vi "Beam_and_Cathode.vi"() -> ()   [LabVIEW 2018]
panel:
  out "?":string
  out "?":string
  out "?":string
  out "?":string
  out "?":string
  out "?":string
  in  "Set Operate Temp C":bool
  out "?":string
  out "?":bool
  out "?":bool
  in  "Set Warm Temp C":bool
  out "?":string
  out "?":string
  out "?":bool
  out "?":bool
  in  "Set Operate Temp B":bool
  out "?":string
  out "?":bool
  out "?":bool
  in  "Set Warm Temp B":bool
  out "?":string
  out "?":string
  out "?":bool
  out "?":bool
  in  "Set Operate Temp A":bool
  out "?":string
  out "?":bool
  out "?":bool
  in  "Set Warm Temp A":bool
  out "?":string
  out "?":string
  out "?":bool
  out "?":bool
  out "Cathode C":string
  out "Cathode B":string
  out "?":string
  out "?":bool
  out "?":bool
  out "?":string
  out "?":bool
  out "?":bool
  out "Cathode A":string
  out "?":string
  out "?":bool
  out "?":bool
  out "?":string
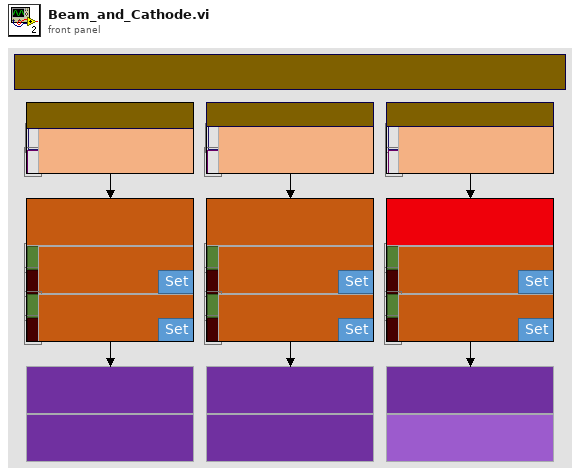
[diagram p1: front panel]
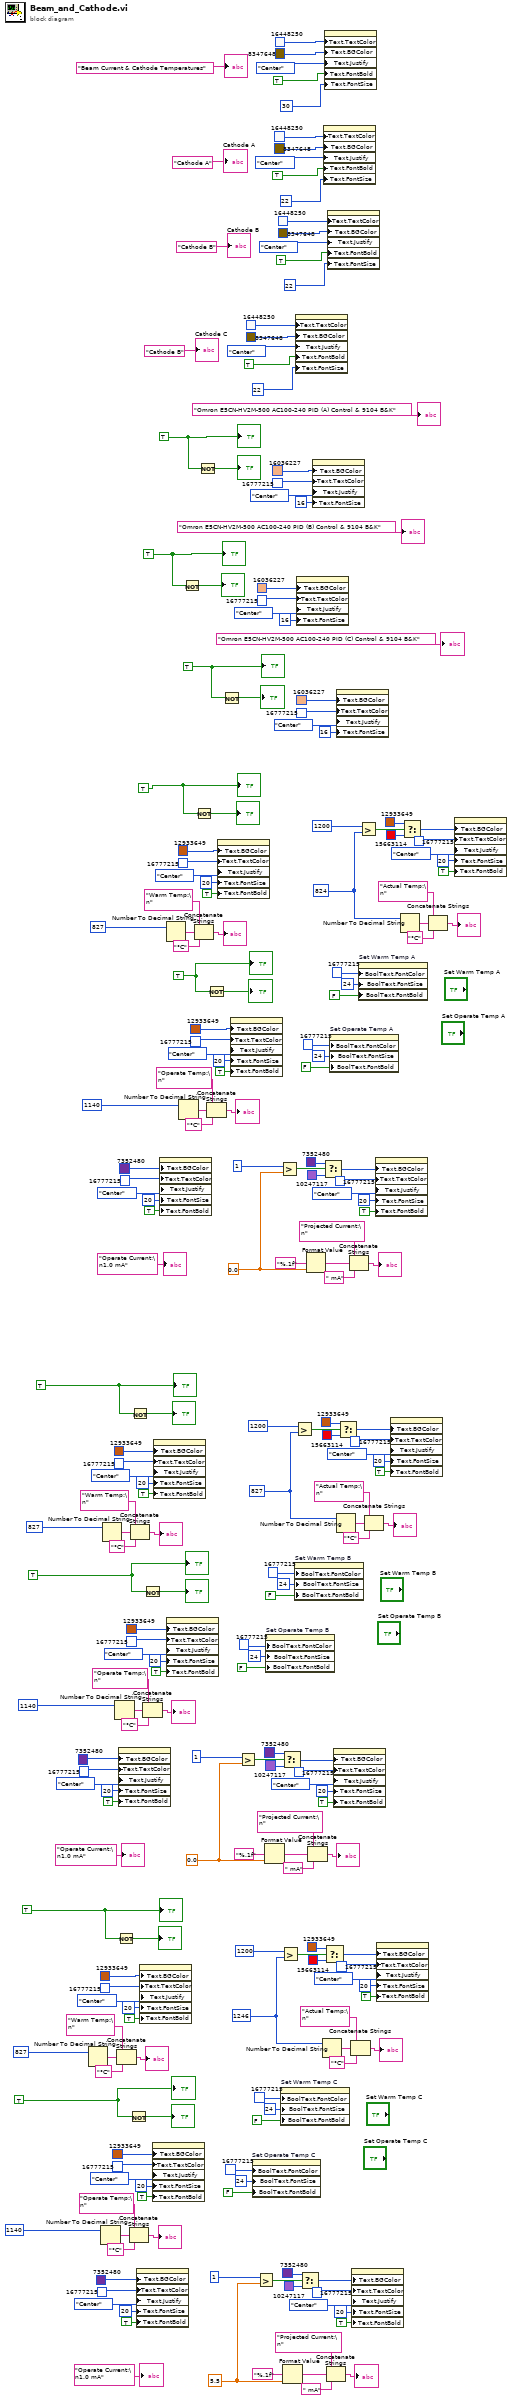
[diagram p0: block diagram]
diagram:
  w1 = 5.5
  w22 = 0.0
  w43 = 0.0
  w64 = TRUE
  w66 = TRUE
  w67 = 1246 ("number")
  w108 = TRUE
  w110 = TRUE
  w111 = 827 ("number")
  w152 = TRUE
  w154 = TRUE
  w155 = 824 ("number")
  w198 = TRUE
  w204 = TRUE
  w211 = TRUE
  n1 = Number To Decimal String(number=827) -> (decimal integer string=w92:string)  [unwired: 1 in]
  n2 = Number To Decimal String(number=1140) -> (decimal integer string=w79:string)  [unwired: 1 in]
  n3 = Number To Decimal String(number=827) -> (decimal integer string=w136:string)  [unwired: 1 in]
  n4 = Number To Decimal String(number=1140) -> (decimal integer string=w123:string)  [unwired: 1 in]
  n5 = Not(x=w64) -> (.not. x?=→"?":bool)
  n6 = Concatenate Strings("Warm Temp:\n", w92, "°C" ("string")) -> (→"?":string)
  n7 = property class="Str"("Text.BGColor"=u32 7352480, "Text.TextColor"=u32 16777215, "Text.Justify"=enum16{"Left", "Center", "Right"}."Center" ("Text.Justification"), "Text.FontSize"=u32 20 ("Text.Font:Size"), "Text.FontBold"=TRUE ("Text.Font:Bold")) -> ()  [unwired: 2 in, 2 out]
  n8 = Not(x=w66) -> (.not. x?=→"?":bool)
  n9 = Concatenate Strings("Operate Temp:\n", w79, "°C" ("string")) -> (→"?":string)
  n10 = Not(x=w108) -> (.not. x?=→"?":bool)
  n11 = Concatenate Strings("Warm Temp:\n", w136, "°C" ("string")) -> (→"?":string)
  n12 = property class="Str"("Text.BGColor"=u32 7352480, "Text.TextColor"=u32 16777215, "Text.Justify"=enum16{"Left", "Center", "Right"}."Center" ("Text.Justification"), "Text.FontSize"=u32 20 ("Text.Font:Size"), "Text.FontBold"=TRUE ("Text.Font:Bold")) -> ()  [unwired: 2 in, 2 out]
  n13 = property class="Str"("Text.BGColor"=u32 12933649, "Text.TextColor"=u32 16777215, "Text.Justify"=enum16{"Left", "Center", "Right"}."Center" ("Text.Justification"), "Text.FontSize"=u32 20 ("Text.Font:Size"), "Text.FontBold"=TRUE ("Text.Font:Bold")) -> ()  [unwired: 2 in, 2 out]
  n14 = Not(x=w110) -> (.not. x?=→"?":bool)
  n15 = Concatenate Strings("Operate Temp:\n", w123, "°C" ("string")) -> (→"?":string)
  n16 = property class="Str"("Text.BGColor"=u32 12933649, "Text.TextColor"=u32 16777215, "Text.Justify"=enum16{"Left", "Center", "Right"}."Center" ("Text.Justification"), "Text.FontSize"=u32 20 ("Text.Font:Size"), "Text.FontBold"=TRUE ("Text.Font:Bold")) -> ()  [unwired: 2 in, 2 out]
  n17 = property class="Str"("Text.BGColor"=u32 12933649, "Text.TextColor"=u32 16777215, "Text.Justify"=enum16{"Left", "Center", "Right"}."Center" ("Text.Justification"), "Text.FontSize"=u32 20 ("Text.Font:Size"), "Text.FontBold"=TRUE ("Text.Font:Bold")) -> ()  [unwired: 2 in, 2 out]
  n18 = property class="Str"("Text.BGColor"=u32 7352480, "Text.TextColor"=u32 16777215, "Text.Justify"=enum16{"Left", "Center", "Right"}."Center" ("Text.Justification"), "Text.FontSize"=u32 20 ("Text.Font:Size"), "Text.FontBold"=TRUE ("Text.Font:Bold")) -> ()  [unwired: 2 in, 2 out]
  n19 = Number To Decimal String(number=827) -> (decimal integer string=w181:string)  [unwired: 1 in]
  n20 = property class="Str"("Text.BGColor"=u32 12933649, "Text.TextColor"=u32 16777215, "Text.Justify"=enum16{"Left", "Center", "Right"}."Center" ("Text.Justification"), "Text.FontSize"=u32 20 ("Text.Font:Size"), "Text.FontBold"=TRUE ("Text.Font:Bold")) -> ()  [unwired: 2 in, 2 out]
  n21 = Number To Decimal String(number=1140) -> (decimal integer string=w168:string)  [unwired: 1 in]
  n22 = Not(x=w204) -> (.not. x?=→"?":bool)
  n23 = Not(x=w152) -> (.not. x?=→"?":bool)
  n24 = Concatenate Strings("Warm Temp:\n", w181, "°C" ("string")) -> (→"?":string)
  n25 = Not(x=w211) -> (.not. x?=→"?":bool)
  n26 = Not(x=w154) -> (.not. x?=→"?":bool)
  n27 = Concatenate Strings("Operate Temp:\n", w168, "°C" ("string")) -> (→"?":string)
  n28 = property class="Str"("Text.BGColor"=u32 12933649, "Text.TextColor"=u32 16777215, "Text.Justify"=enum16{"Left", "Center", "Right"}."Center" ("Text.Justification"), "Text.FontSize"=u32 20 ("Text.Font:Size"), "Text.FontBold"=TRUE ("Text.Font:Bold")) -> ()  [unwired: 2 in, 2 out]
  n29 = Not(x=w198) -> (.not. x?=→"?":bool)
  n30 = property class="Str"("Text.BGColor"=u32 12933649, "Text.TextColor"=u32 16777215, "Text.Justify"=enum16{"Left", "Center", "Right"}."Center" ("Text.Justification"), "Text.FontSize"=u32 20 ("Text.Font:Size"), "Text.FontBold"=TRUE ("Text.Font:Bold")) -> ()  [unwired: 2 in, 2 out]
  n31 = Greater?(x=1, y=w22) -> (0:w27:bool)
  n32 = property on="Set Operate Temp C" class="Bool (strict)"("BoolText.FontColor"=u32 16777215, "BoolText.FontSize"=u32 24 ("Boolean Text.Font:Size"), "BoolText.FontBold"=FALSE ("Boolean Text.Font:Bold")) -> ()  [unwired: 2 in, 2 out]
  n33 = Greater?(x=1, y=w1) -> (0:w6:bool)
  n34 = Format Value(format string="%.1f", value (0)=w22) -> (output string=w23:string)  [unwired: 1 in]
  n35 = property on="Set Operate Temp B" class="Bool (strict)"("BoolText.FontColor"=u32 16777215, "BoolText.FontSize"=u32 24 ("Boolean Text.Font:Size"), "BoolText.FontBold"=FALSE ("Boolean Text.Font:Bold")) -> ()  [unwired: 2 in, 2 out]
  n36 = Greater?(x=1, y=w43) -> (0:w48:bool)
  n37 = Greater?(x=1200, y=w67) -> (0:w68:bool)
  n38 = property on="Set Warm Temp C" class="Bool (strict)"("BoolText.FontColor"=u32 16777215, "BoolText.FontSize"=u32 24 ("Boolean Text.Font:Size"), "BoolText.FontBold"=FALSE ("Boolean Text.Font:Bold")) -> ()  [unwired: 2 in, 2 out]
  n39 = Select(t=u32 7352480, s=w27, f=u32 10247117) -> (s? t:f=w29:u32)
  n40 = Format Value(format string="%.1f", value (0)=w1) -> (output string=w2:string)  [unwired: 1 in]
  n41 = Greater?(x=1200, y=w111) -> (0:w112:bool)
  n42 = property on="Set Warm Temp B" class="Bool (strict)"("BoolText.FontColor"=u32 16777215, "BoolText.FontSize"=u32 24 ("Boolean Text.Font:Size"), "BoolText.FontBold"=FALSE ("Boolean Text.Font:Bold")) -> ()  [unwired: 2 in, 2 out]
  n43 = property on="Cathode C" class="Str"("Text.TextColor"=u32 16448250, "Text.BGColor"=u32 8347648, "Text.Justify"=enum16{"Left", "Center", "Right"}."Center" ("Text.Justification"), "Text.FontBold"=TRUE ("Text.Font:Bold"), "Text.FontSize"=u32 22 ("Text.Font:Size")) -> ()  [unwired: 2 in, 2 out]
  n44 = property class="Str"("Text.BGColor"=u32 16036227, "Text.TextColor"=u32 16777215, "Text.Justify"=enum16{"Left", "Center", "Right"}."Center" ("Text.Justification"), "Text.FontSize"=u32 16 ("Text.Font:Size")) -> ()  [unwired: 2 in, 2 out]
  n45 = Select(t=u32 7352480, s=w6, f=u32 10247117) -> (s? t:f=w8:u32)
  n46 = Format Value(format string="%.1f", value (0)=w43) -> (output string=w44:string)  [unwired: 1 in]
  n47 = Concatenate Strings("Projected Current:\n", w23, " mA" ("string")) -> (→"?":string)
  n48 = property class="Str"("Text.BGColor"=u32 16036227, "Text.TextColor"=u32 16777215, "Text.Justify"=enum16{"Left", "Center", "Right"}."Center" ("Text.Justification"), "Text.FontSize"=u32 16 ("Text.Font:Size")) -> ()  [unwired: 2 in, 2 out]
  n49 = Number To Decimal String(number=w67) -> (decimal integer string=w101:string)  [unwired: 1 in]
  n50 = property on="Cathode A" class="Str"("Text.TextColor"=u32 16448250, "Text.BGColor"=u32 8347648, "Text.Justify"=enum16{"Left", "Center", "Right"}."Center" ("Text.Justification"), "Text.FontBold"=TRUE ("Text.Font:Bold"), "Text.FontSize"=u32 22 ("Text.Font:Size")) -> ()  [unwired: 2 in, 2 out]
  n51 = Select(t=u32 7352480, s=w48, f=u32 10247117) -> (s? t:f=w50:u32)
  n52 = property class="Str"("Text.TextColor"=u32 16448250, "Text.BGColor"=u32 8347648, "Text.Justify"=enum16{"Left", "Center", "Right"}."Center" ("Text.Justification"), "Text.FontBold"=TRUE ("Text.Font:Bold"), "Text.FontSize"=u32 30 ("Text.Font:Size")) -> ()  [unwired: 2 in, 2 out]
  n53 = Select(t=u32 12933649, s=w68, f=u32 15663114) -> (s? t:f=w70:u32)
  n54 = Concatenate Strings("Projected Current:\n", w2, " mA" ("string")) -> (→"?":string)
  n55 = property on="Cathode B" class="Str"("Text.TextColor"=u32 16448250, "Text.BGColor"=u32 8347648, "Text.Justify"=enum16{"Left", "Center", "Right"}."Center" ("Text.Justification"), "Text.FontBold"=TRUE ("Text.Font:Bold"), "Text.FontSize"=u32 22 ("Text.Font:Size")) -> ()  [unwired: 2 in, 2 out]
  n56 = property on="Set Operate Temp A" class="Bool (strict)"("BoolText.FontColor"=u32 16777215, "BoolText.FontSize"=u32 24 ("Boolean Text.Font:Size"), "BoolText.FontBold"=FALSE ("Boolean Text.Font:Bold")) -> ()  [unwired: 2 in, 2 out]
  n57 = property class="Str"("Text.BGColor"=w29, "Text.TextColor"=u32 16777215, "Text.Justify"=enum16{"Left", "Center", "Right"}."Center" ("Text.Justification"), "Text.FontSize"=u32 20 ("Text.Font:Size"), "Text.FontBold"=TRUE ("Text.Font:Bold")) -> ()  [unwired: 2 in, 2 out]
  n58 = property class="Str"("Text.BGColor"=u32 16036227, "Text.TextColor"=u32 16777215, "Text.Justify"=enum16{"Left", "Center", "Right"}."Center" ("Text.Justification"), "Text.FontSize"=u32 16 ("Text.Font:Size")) -> ()  [unwired: 2 in, 2 out]
  n59 = Number To Decimal String(number=w111) -> (decimal integer string=w145:string)  [unwired: 1 in]
  n60 = Select(t=u32 12933649, s=w112, f=u32 15663114) -> (s? t:f=w114:u32)
  n61 = Concatenate Strings("Projected Current:\n", w44, " mA" ("string")) -> (→"?":string)
  n62 = Concatenate Strings("Actual Temp:\n", w101, "°C" ("string")) -> (→"?":string)
  n63 = property class="Str"("Text.BGColor"=w8, "Text.TextColor"=u32 16777215, "Text.Justify"=enum16{"Left", "Center", "Right"}."Center" ("Text.Justification"), "Text.FontSize"=u32 20 ("Text.Font:Size"), "Text.FontBold"=TRUE ("Text.Font:Bold")) -> ()  [unwired: 2 in, 2 out]
  n64 = Greater?(x=1200, y=w155) -> (0:w156:bool)
  n65 = property on="Set Warm Temp A" class="Bool (strict)"("BoolText.FontColor"=u32 16777215, "BoolText.FontSize"=u32 24 ("Boolean Text.Font:Size"), "BoolText.FontBold"=FALSE ("Boolean Text.Font:Bold")) -> ()  [unwired: 2 in, 2 out]
  n66 = Concatenate Strings("Actual Temp:\n", w145, "°C" ("string")) -> (→"?":string)
  n67 = property class="Str"("Text.BGColor"=w50, "Text.TextColor"=u32 16777215, "Text.Justify"=enum16{"Left", "Center", "Right"}."Center" ("Text.Justification"), "Text.FontSize"=u32 20 ("Text.Font:Size"), "Text.FontBold"=TRUE ("Text.Font:Bold")) -> ()  [unwired: 2 in, 2 out]
  n68 = property class="Str"("Text.BGColor"=w70, "Text.TextColor"=u32 16777215, "Text.Justify"=enum16{"Left", "Center", "Right"}."Center" ("Text.Justification"), "Text.FontSize"=u32 20 ("Text.Font:Size"), "Text.FontBold"=TRUE ("Text.Font:Bold")) -> ()  [unwired: 2 in, 2 out]
  n69 = property class="Str"("Text.BGColor"=w114, "Text.TextColor"=u32 16777215, "Text.Justify"=enum16{"Left", "Center", "Right"}."Center" ("Text.Justification"), "Text.FontSize"=u32 20 ("Text.Font:Size"), "Text.FontBold"=TRUE ("Text.Font:Bold")) -> ()  [unwired: 2 in, 2 out]
  n70 = Number To Decimal String(number=w155) -> (decimal integer string=w190:string)  [unwired: 1 in]
  n71 = Select(t=u32 12933649, s=w156, f=u32 15663114) -> (s? t:f=w158:u32)
  n72 = Concatenate Strings("Actual Temp:\n", w190, "°C" ("string")) -> (→"?":string)
  n73 = property class="Str"("Text.BGColor"=w158, "Text.TextColor"=u32 16777215, "Text.Justify"=enum16{"Left", "Center", "Right"}."Center" ("Text.Justification"), "Text.FontSize"=u32 20 ("Text.Font:Size"), "Text.FontBold"=TRUE ("Text.Font:Bold")) -> ()  [unwired: 2 in, 2 out]
  "?" <- "Beam Current & Cathode Temperatures" ("String")
  "Cathode A" <- "Cathode A" ("String")
  "Cathode B" <- "Cathode B" ("String")
  "Cathode C" <- "Cathode B" ("String")
  "?" <- w211
  "?" <- "Omron E5CN-HV2M-500 AC100-240 PID (A) Control & 9104 B&K"
  "?" <- w204
  "?" <- "Omron E5CN-HV2M-500 AC100-240 PID (B) Control & 9104 B&K"
  "?" <- w198
  "?" <- "Omron E5CN-HV2M-500 AC100-240 PID (C) Control & 9104 B&K"
  "?" <- w152
  "?" <- w154
  "?" <- w108
  "?" <- w110
  "?" <- w64
  "?" <- w66
  "?" <- "Operate Current:\n1.0 mA"
  "?" <- "Operate Current:\n1.0 mA"
  "?" <- "Operate Current:\n1.0 mA"
